vi "DataStorageDataSetPacketRoutedMessage_Parse.vi"(8 "error in (no error)":errorcluster, 11 "Message":T5) -> (0 "error out":errorcluster, 1 "DataSet":T4, 2 "Header":T2, 3 "DataStorageDataSetPacketRoutedMessage":T1)   [LabVIEW 2017]
uses:
  <vilib>/addons/InsightCM/MessageBus/Base/controls/Message.ctl
  <vilib>/addons/InsightCM/MessageBus/Base/controls/MessageHeader.ctl
  <vilib>/addons/InsightCM/MessageBus/Base/controls/KeyValuePair.ctl
  <vilib>/addons/InsightCM/MessageBus/Base/controls/DataSetPacket.ctl
  <vilib>/addons/InsightCM/MessageBus/MessageLibrary/DataStorage/controls/DataStorageDataSetPacketRoutedMessage.ctl
  <vilib>/addons/InsightCM/Utilities/PropertyHelpers/PropertyHelpers.lvlib
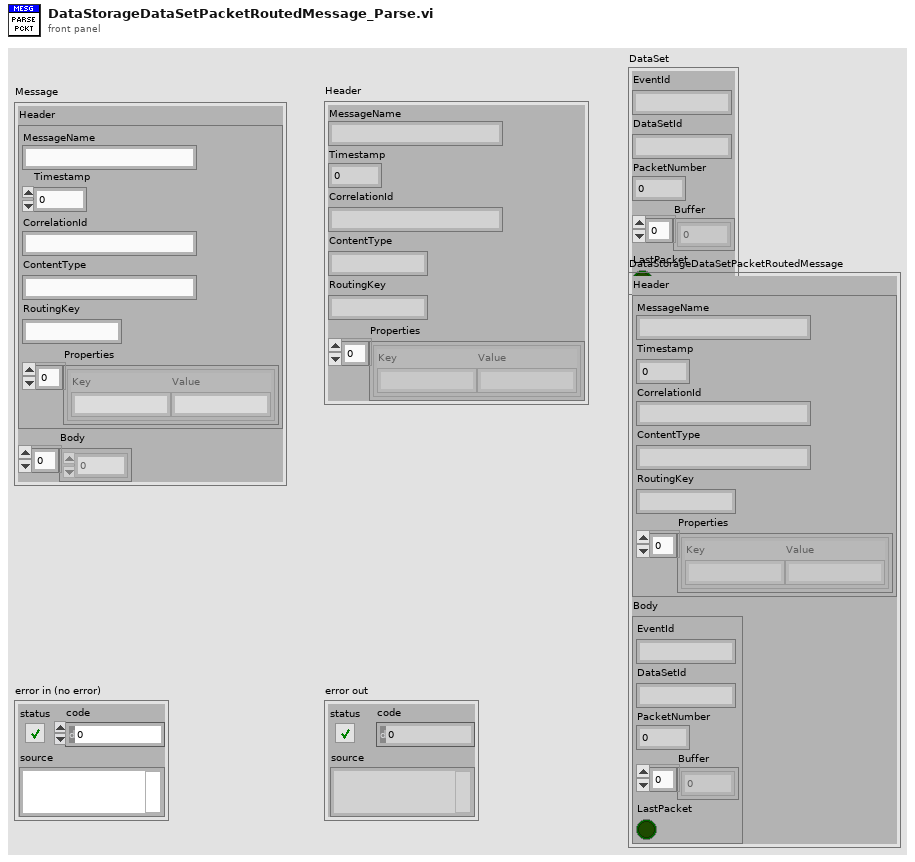
[diagram p1: front panel]
types:
  T1 = typedef "DataStorageDataSetPacketRoutedMessage.ctl" = cluster{"Header":T2, "Body":T4}
  T2 = typedef "MessageHeader.ctl" = cluster{"MessageName":string, "Timestamp":i64, "CorrelationId":string, "ContentType":string, "RoutingKey":string, "Properties":T3[]}
  T3 = typedef "KeyValuePair.ctl" = cluster{"Key":string, "Value":string}
  T4 = typedef "DataSetPacket.ctl" = cluster{"EventId":string, "DataSetId":string, "PacketNumber":i32, "Buffer":u8[], "LastPacket":bool}
  T5 = typedef "Message.ctl" = cluster{"Header":T2, "Body":u8[]}
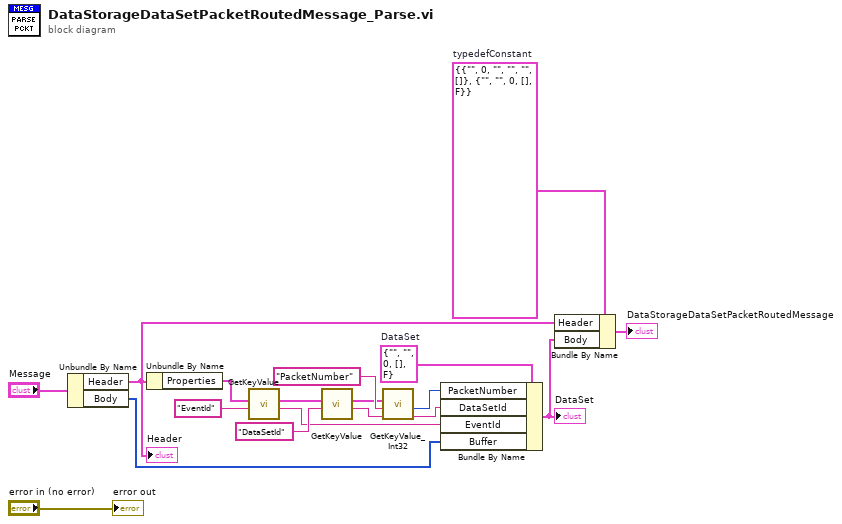
[diagram p0: block diagram]
diagram:
  w14 = T1 {"Header"={"MessageName"="", "Timestamp"=0, "CorrelationId"="", "ContentType"="", "RoutingKey"="", "Properties"=[]}, "Body"={"EventId"="", "DataSetId"="", "PacketNumber"=0, "Buffer"=[], "LastPacket"=FALSE}}  # typedefConstant
  w7 = T4 {"EventId"="", "DataSetId"="", "PacketNumber"=0, "Buffer"=[], "LastPacket"=FALSE}  # DataSet
  n1 = Unbundle By Name("Message") -> ("Header"=w16:T2, "Body"=w12:u8[])
  "Header" <- w16
  n2 = Unbundle By Name(w16) -> ("Properties"=w11:T3[])
  n3 = call <vilib>:"GetKeyValue.vi"("key"="EventId" ("Key"), "key value pairs"=w11) -> ("value"=w2:string, "key value pairs out"=w5:T3[])  [unwired: 7 in, 1 out]
  n4 = call <vilib>:"GetKeyValue.vi"("key"="DataSetId" ("Key"), "key value pairs"=w5) -> ("value"=w1:string, "key value pairs out"=w4:T3[])  [unwired: 7 in, 1 out]
  n5 = call <vilib>:"GetKeyValue_Int32.vi"("key"="PacketNumber" ("Key"), "key value pairs"=w4) -> ("value"=w9:i32)  [unwired: 7 in, 2 out]
  n6 = Bundle By Name(cluster=w7, "PacketNumber"=w9, "DataSetId"=w1, "EventId"=w2, "Buffer"=w12) -> (w13:T4)
  "DataSet" <- w13
  n7 = Bundle By Name(cluster=w14, "Header"=w16, "Body"=w13) -> (→"DataStorageDataSetPacketRoutedMessage":T1)
  "error out" <- "error in (no error)"
